vi "Renishaw-XL80_GetLambda.vi"(8 "error in (no error)":errorcluster, 11 "Renishaw-XL80_EMU in":refnum<class "Renishaw-XL80_EMU.lvclass">) -> (0 "error out":errorcluster, 2 "Lambda":dbl, 3 "Renishaw-XL80_EMU out":refnum<class "Renishaw-XL80_EMU.lvclass">)   [LabVIEW 2024, in "Renishaw-XL80_EMU.lvclass"]
doc: "Reading this property retrieves the current wavelength in µm.\n\nDefinition\nHRESULTget_Lambda( [out, retval] double* pVal);\nParameters\npVal\nA variable that will be set to the current wavelength (in µm).\n\nComments\nReading this property will always retrieve the current wavelength (provided pVal is a valid pointer).\n\nThe property will normally return an HRESULT of S_OK. However, it will return E_POINTER if the client supplies a null pointer for pVal."
uses:
  Renishaw-XL80_EMU.lvclass
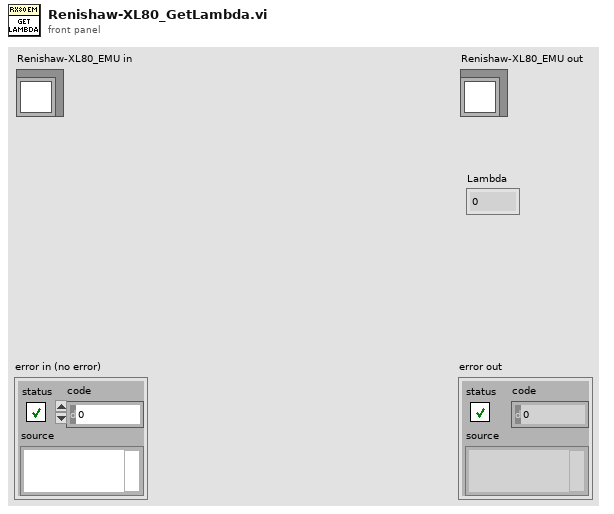
[diagram p1: front panel]
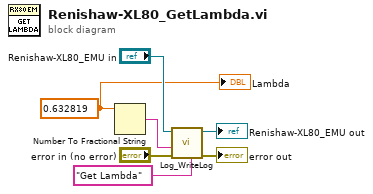
[diagram p0: block diagram]
diagram:
  w3 = 0.632819 ("Lambda")
  n1 = Number To Fractional String(number=w3) -> (F-format string=w2:string)  [unwired: 3 in]
  n2 = call-dynamic "Log_WriteLog.vi"("Additional text"="Get Lambda", "error in (no error)"="error in (no error)", "Response"=w2, "Log in"="Renishaw-XL80_EMU in") -> ("error out"=→"error out":errorcluster, "Log out"=→"Renishaw-XL80_EMU out":refnum<class "Renishaw-XL80_EMU.lvclass">)  [unwired: 6 in]
  "Lambda" <- w3
